vi "ITC503 Connect.vi"(0 "ITC Selector":u16(ring) items=["ITC503s"]) -> (1 "ITC Setup":T1={"Description"="", "IO Info"={"Address"={"Com Port"=1, "ISOBUS Address"=1, "GPIB Address"=24, "Communication"=enum."ISOBUS"}, "Version"=enum."ITC503", "Ch 1 dec places"=1, "Ch 2 dec places"=1, "Ch 3 dec places"=1, "Ch1 Name"="", "Ch2 Name"="", "Ch3 Name"=""}}, 2 "Connected":bool)   [LabVIEW 2010]
uses:
  drivers/Oxford ITC/ITCAPPS.LLB/ITCSetup.ctl
  drivers/Oxford ITC/ITCSUBS.LLB/ITCIO.ctl
  drivers/Oxford ITC/BUSGEN.LLB/OxfordAddress.ctl
  drivers/Oxford ITC/ITCSUBS.LLB/ITCVersion.ctl
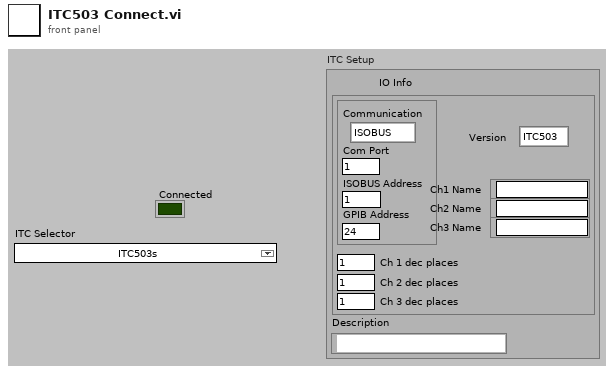
[diagram p1: front panel]
types:
  T1 = typedef "ITCSetup.ctl" = cluster{"Description":string, "IO Info":T2}
  T2 = typedef "ITCIO.ctl" = cluster{"Address":T3, "Version":T4, "Ch 1 dec places":i16, "Ch 2 dec places":i16, "Ch 3 dec places":i16, "Ch1 Name":string, "Ch2 Name":string, "Ch3 Name":string}
  T3 = typedef "OxfordAddress.ctl" = cluster{"Com Port":i32, "ISOBUS Address":i32, "GPIB Address":i16, "Communication":enum16{"RS232", "ISOBUS", "GPIB", "Gateway"}}
  T4 = typedef "ITCVersion.ctl" = enum16{"ITC502", "ITC503", "ITC601"}
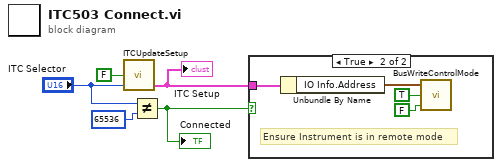
[diagram p0: block diagram]
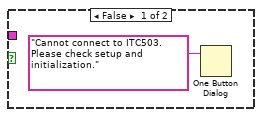
[diagram p2: hidden frame]
diagram:
  n1 = call "ITCUpdateSetup.vi"("Index"="ITC Selector", "Write to disk?"=FALSE) -> ("ITC Setup"=w3:T1)  [unwired: 2 in, 1 out]
  "ITC Setup" <- w3
  n2 = Not Equal?(x="ITC Selector", y=65536) -> (x != y?=w4:bool)
  "Connected" <- w4
  n3 = case shown="True" w4 {
    tunnel: w3 -> [_ w7]
    frame False {
      n4 = One Button Dialog(message="Cannot connect to ITC503. Please check setup and initialization.") -> ()  [unwired: 1 in, 1 out]
    }
    frame True {
      # "Ensure Instrument is in remote mode"
      n5 = Unbundle By Name(w7) -> ("IO Info.Address"=w10:T3)
      n6 = call "BusWriteControlMode.vi"("Locked"=FALSE, "Remote"=TRUE, "Address"=w10) -> ()  [unwired: 1 out]
    }
  }
